vi "Process.vi"(8 "error in (no error)":errorcluster, 10 "Pound in":refnum<class "Pound.lvclass">, 11 "Qbus in":refnum<class "Qbus.lvclass">) -> (0 "error out":errorcluster)   [LabVIEW 2017, in "IrAcquisition.lvlib"]
uses:
  <vilib>/addons/InsightCM/Devices/Shared/Ir/IrAcquisition/IrAcquisition.lvlib
  <vilib>/addons/Qbus/Qbus.lvclass
  <vilib>/NI/Software Watchdog/Pound/Pound.lvclass
  <vilib>/addons/InsightCM/Devices/Shared/Ir/IrAcquisition/controls/config.ctl
  <vilib>/addons/InsightCM/Devices/Shared/Ir/IrAcquisition/controls/camera.ctl
  <vilib>/userdefined/High Color/IMAQdx.ctl
  <vilib>/vision/Image Controls.llb/IMAQ Image.ctl
  <vilib>/addons/PointValueMap/controls/PointMap.ctl
  <vilib>/addons/TimerProcess/controls/taskType.ctl
  <vilib>/addons/InsightCM/Devices/Shared/Ir/IrManageCameras/controls/camera.ctl
  <vilib>/addons/InsightCM/Devices/Shared/Common/DataFlow/controls/Type.ctl
  <vilib>/addons/TraceLogger/TraceLogger.lvlib
  <vilib>/NI/Software Watchdog/Watchdog/Watchdog.lvclass
  <vilib>/addons/InsightCM/Devices/Shared/Ir/IrManageCameras/IrManageCameras.lvlib
  <vilib>/addons/TimerProcess/TimerProcess.lvlib
  <vilib>/addons/InsightCM/Devices/Shared/Common/DataFlow/DataFlow.lvlib
  <vilib>/addons/PointValueMap/PointValueMap.lvlib
  <vilib>/addons/InsightCM/Devices/Shared/Ir/IrDataEventCreator/IrDataEventCreator.lvlib
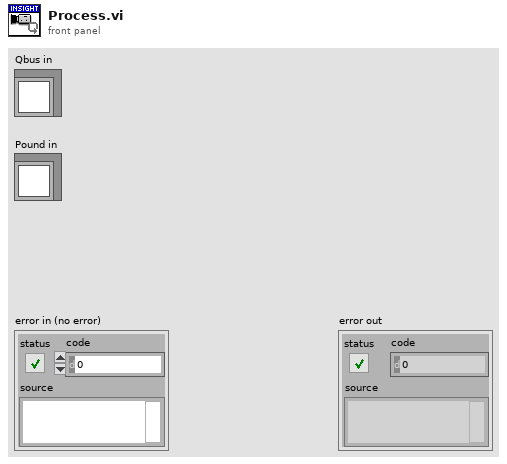
[diagram p1: front panel]
types:
  T1 = typedef "IrAcquisition.lvlib/config.ctl" = cluster{"active cameras":T2[], "poll interval (sec)":dbl}
  T2 = typedef "IrAcquisition.lvlib/camera.ctl" = cluster{"Name":string, "ChannelId":string, "CameraId":string, "SerialNumber":string, "Unit":string, "IMAQSession":T3, "InterfaceName":string, "RawImage":T4, "ScaledImage":T4, "TestPanelImage":T4, "Map":T5, "InDeviceModel":bool}
  T3 = typedef "IMAQdx.ctl" = refnum<k21>
  T4 = typedef "IMAQ Image.ctl" = refnum<image>
  T5 = typedef "PointValueMap.lvlib/PointMap.ctl" = refnum<data-value>
  T6 = typedef "TimerProcess.lvlib/taskType.ctl" = enum16{"single", "repeat"}
  T7 = typedef "IrManageCameras.lvlib/camera.ctl" = cluster{"InterfaceName":string, "VendorName":string, "ModelName":string, "CameraFileName":string, "SerialNumber":string, "IP Address":string, "PhysicalPort":string, "CameraName":string, "ChannelId":string, "CameraId":string, "InDeviceModel":bool}
  T8 = typedef "DataFlow.lvlib/Type.ctl" = enum16{"High Rate", "Low Rate", "Burst Mode"}
  T9 = typedef "IrDataEventCreator.lvlib/RegisterImageRoutedMessage.ctl" = cluster{"Name":string, "Image Registry":T10}
  T10 = typedef "IrDataEventCreator.lvlib/Registry_Image.ctl" = cluster{"Properties":T11[]}
  T11 = typedef "KeyValuePair.ctl" = cluster{"Key":string, "Value":string}
  T12 = typedef "DataFlow.lvlib/Data.ctl" = cluster{"DataGroup":string, "Waveforms":T13, "Map":T5, "Type":T8}
  T13 = typedef "wfmSGL_DVR.ctl" = refnum<data-value>
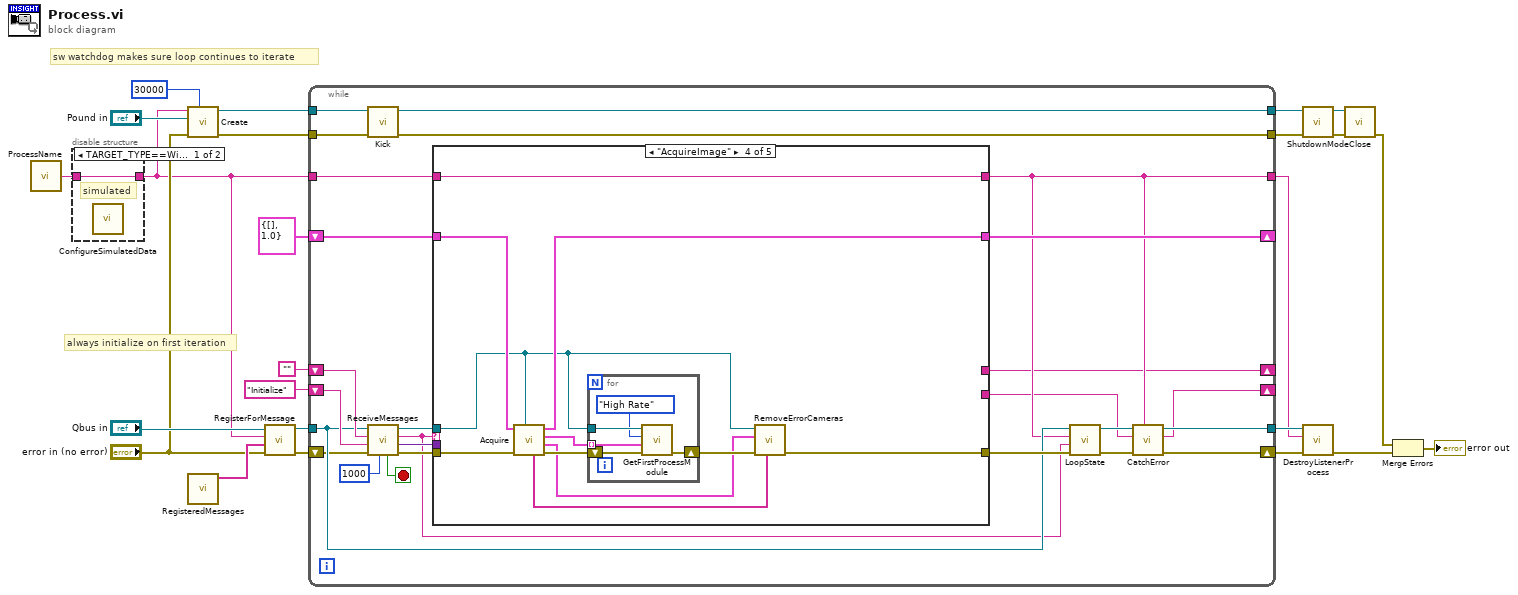
[diagram p0: block diagram]
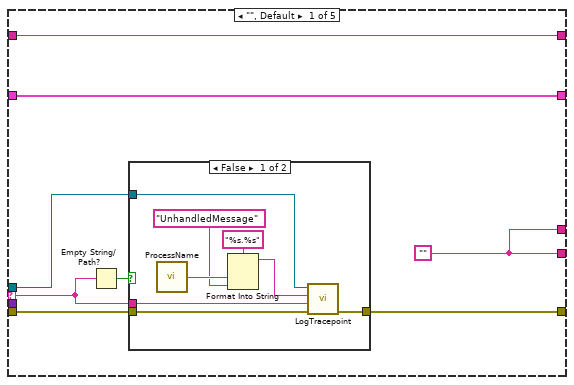
[diagram p3: hidden frame]
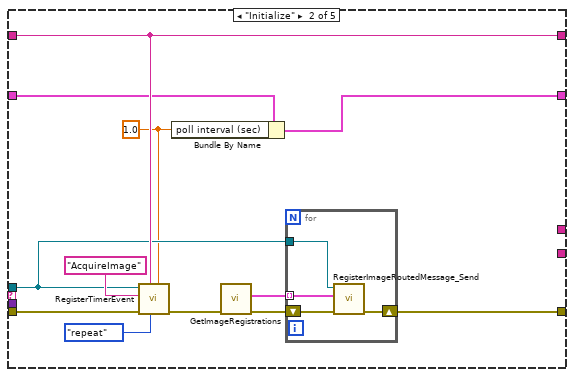
[diagram p5: hidden frame]
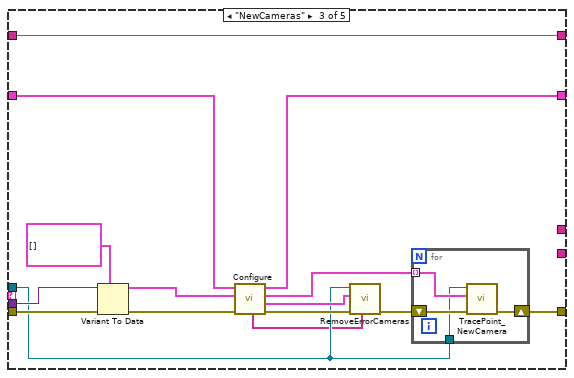
[diagram p6: hidden frame]
diagram:
  # "always initialize on first iteration"
  # "sw watchdog makes sure loop continues to iterate"
  n1 = call <vilib>:"ProcessName.vi"() -> ("process name"=w1:string)  [unwired: 5 in]
  n2 = disable-structure shown="TARGET_TYPE==Windows" {
    disable-tunnel: [w25 w26] -> w2
    disable-tunnel: w1 -> [w25 w26]
    frame condition #0 (active) {
      # "simulated"
      n3 = call <vilib>:"ConfigureSimulatedData.vi"() -> ()  [unwired: 12 in]
    }
    frame condition #1 {
    }
  }
  n4 = call <vilib>:"Create.vi"("Execution Timeout (ms)"=u32 30000, "error in (no error)"="error in (no error)", "Pound"="Pound in", "Name"=w2) -> ("error out"=w8:errorcluster, "Watchdog"=w14:refnum<data-value>)  [unwired: 6 in]
  n5 = call <vilib>:"RegisteredMessages.vi"() -> ("registered messages"=w15:string[])  [unwired: 11 in]
  n6 = call <vilib>:"RegisterForMessage.vi"("error in (no error)"="error in (no error)", "message names"=w15, "process name"=w2, "Qbus in"="Qbus in") -> ("error in (no error)"=w23:errorcluster, "Qbus out"=w22:refnum<class "Qbus.lvclass">)  [unwired: 6 in]
  n7 = while {
    shift-right: [w27] -> _
    shift-left: "" -> [w51]
    tunnel: w22 -> [w40]
    tunnel: w2 -> [w30]
    tunnel: [w43] -> w20
    tunnel: [w29] -> w19
    shift-right: [w42] -> _
    shift-left: "Initialize" -> [w47]
    shift-right: [w45] -> _
    shift-left: T1 {"active cameras"=[], "poll interval (sec)"=1.0} ("config") -> [w46]
    tunnel: w14 -> [w39]
    tunnel: [w38] -> w10
    tunnel: w8 -> [w37]
    tunnel: [w35] -> w7
    shift-right: [w44] -> w21
    shift-left: w23 -> [w36]
    stop <- w52 stop-if-true
    n8 = call <vilib>:"Kick.vi"("error in (no error)"=w37, "Watchdog"=w39) -> ("error out"=w35:errorcluster, "Watchdog"=w38:refnum<data-value>)  [unwired: 8 in]
    n9 = call <vilib>:"ReceiveMessages.vi"("Timeout(1000)"=1000 ("milliseconds to wait"), "error in (no error)"=w36, "priority action"=w47, "default action"=w51, "Qbus in"=w40) -> ("error out"=w50:errorcluster, "message value"=w48:variant, "action"=w34:string, "Qbus out"=w49:refnum<class "Qbus.lvclass">, "exit"=w52:bool)  [unwired: 2 in]
    n10 = case shown="\"AcquireImage\"" w34 {
      selector: w34 -> [w56 _ _ _ _]
      tunnel: w50 -> [w58 w81 w99 w114 w123]
      tunnel: w49 -> [w54 w77 w88 w105 _]
      tunnel: [w57 w70 w87 w108 w123] -> w41
      tunnel: w48 -> [_ _ w98 _ _]
      tunnel: w46 -> [w60 w73 w94 w112 w122]
      tunnel: [w60 w72 w93 w111 w122] -> w45
      tunnel: [w59 w79 w100 w115 w121] -> w29
      tunnel: w30 -> [w59 w79 w100 w115 w121]
      tunnel: [w53 _ _ _ _] -> w28
      tunnel: [w53 _ _ _ _] -> w27
      frame "", Default {
        w53 = ""
        n11 = Empty String/Path?(string/path=w56) -> (empty?=w55:bool)
        n12 = case shown="False" w55 {
          tunnel: [w67 w69] -> w57
          tunnel: w58 -> [w68 w69]
          tunnel: w56 -> [w65 _]
          tunnel: w54 -> [w66 _]
          frame False {
            n13 = call <vilib>:"ProcessName.vi"() -> ("process name"=w63:string)  [unwired: 5 in]
            n14 = Format Into String(format string="%s.%s", w63, "UnhandledMessage" ("ProcessName")) -> (resulting string=w61:string)  [unwired: 2 in, 1 out]
            n15 = call <vilib>:"LogTracepoint.vi"("error in (no error)"=w68, "log string"=w65, "tracepoint"=w61, "qbus in"=w66) -> ("error out"=w67:errorcluster)  [unwired: 6 in, 1 out]
          }
          frame True {
          }
        }
      }
      frame "Initialize" {
        w71 = 1.0 ("interval (sec)")
        n16 = call <vilib>:"RegisterTimerEvent.vi"("interval (sec)"=w71, "type"=taskType."repeat", "process name"=w79, "error in (no error)"=w81, "callback action"="AcquireImage", "qbus in"=w77) -> ("error out"=w76:errorcluster)  [unwired: 4 in, 1 out]
        n17 = Bundle By Name(cluster=w73, "poll interval (sec)"=w71) -> (w72:T1)
        n18 = call <vilib>:"GetImageRegistrations.vi"("error in (no error)"=w76) -> ("error out"=w75:errorcluster, "RegisterImage"=w74:T9[])  [unwired: 9 in]
        n19 = for {
          tunnel: w77 -> [w82]
          shift-right: [w83] -> w70
          shift-left: w75 -> [w84]
          tunnel: w74 -> [w85] mode=indexing
          n20 = call <vilib>:"RegisterImageRoutedMessage_Send.vi"("error in (no error)"=w84, "RegisterImageRoutedMessage"=w85, "Qbus in"=w82) -> ("error out"=w83:errorcluster)  [unwired: 7 in, 1 out]
        }
      }
      frame "NewCameras" {
        n21 = Variant To Data(error in=w99, type=T7[] [] ("new cameras"), Variant=w98) -> (data=w95:T7[], error out=w96:errorcluster)
        n22 = call <vilib>:"Configure.vi"("error in (no error)"=w96, "new cameras"=w95, "config"=w94) -> ("error out"=w92:errorcluster, "error cameras"=w91:T2[], "new cameras"=w90:T2[], "config out"=w93:T1, "error text"=w86:string[])  [unwired: 4 in]
        n23 = call <vilib>:"RemoveErrorCameras.vi"("error text"=w86, "error in (no error)"=w92, "error cameras"=w91, "Qbus in"=w88) -> ("error out"=w89:errorcluster)  [unwired: 7 in]
        n24 = for {
          tunnel: w90 -> [w104] mode=indexing
          shift-right: [w102] -> w87
          shift-left: w89 -> [w103]
          tunnel: w88 -> [w101]
          n25 = call <vilib>:"TracePoint_NewCamera.vi"("error in (no error)"=w103, "new camera"=w104, "Qbus"=w101) -> ("error out"=w102:errorcluster)  [unwired: 8 in]
        }
      }
      frame "AcquireImage" {
        n26 = call <vilib>:"Acquire.vi"("Qbus"=w105, "error in (no error)"=w114, "config"=w112) -> ("error out"=w113:errorcluster, "error cameras"=w107:T2[], "new data"=w110:T12[], "config out"=w111:T1, "error text"=w106:string[])  [unwired: 4 in]
        n27 = for {
          shift-right: [w119] -> w109
          shift-left: w113 -> [w120]
          tunnel: w105 -> [w118]
          tunnel: w110 -> [w117] mode=indexing
          n28 = call <vilib>:"GetFirstProcessModule.vi"("error in (no error)"=w120, "data"=w117, "type"=Type."High Rate", "Qbus in"=w118) -> ("error out"=w119:errorcluster)  [unwired: 6 in, 1 out]
        }
        n29 = call <vilib>:"RemoveErrorCameras.vi"("error text"=w106, "error in (no error)"=w109, "error cameras"=w107, "Qbus in"=w105) -> ("error out"=w108:errorcluster)  [unwired: 7 in]
      }
      frame "Exit" {
      }
    }
    n30 = call <vilib>:"LoopState.vi"("error in (no error)"=w41, "loop action"=w34, "process name"=w29, "Qbus in"=w40) -> ("error out"=w32:errorcluster, "Qbus out"=w31:refnum<class "Qbus.lvclass">)  [unwired: 6 in]
    n31 = call <vilib>:"CatchError.vi"("source"=w29, "error in (no error)"=w32, "next action in"=w28, "Qbus in"=w31) -> ("error out"=w44:errorcluster, "next action out"=w42:string, "Qbus out"=w43:refnum<class "Qbus.lvclass">)  [unwired: 5 in]
  }
  n32 = call <vilib>:"ShutdownMode.vi"("error in (no error)"=w7, "Watchdog"=w10) -> ("error out"=w9:errorcluster, "Watchdog"=w11:refnum<data-value>)  [unwired: 8 in]
  n33 = call <vilib>:"DestroyListenerProcess.vi"("error in (no error)"=w21, "process name"=w19, "Qbus in"=w20) -> ("error in (no error)"=w6:errorcluster)  [unwired: 7 in, 1 out]
  n34 = call <vilib>:"Close.vi"("error in (no error)"=w9, "Watchdog"=w11) -> ("error out"=w5:errorcluster)  [unwired: 9 in]
  n35 = Merge Errors(w5, w6) -> (→"error out":errorcluster)
